vi "GIS Error Monitor Process.vi"(8 "error in":errorcluster, 9 "notifierSync":refnum<notifier>, 10 "TopLevel":refnum<class "TopLevel.lvclass">, 11 "GIS Printer in":refnum<class "GIS Printer.lvclass">) -> (3 "GIS Printer out":refnum<class "GIS Printer.lvclass">)   [LabVIEW 2022 SP3, in "GIS Printer.lvclass"]
uses:
  GIS Printer.lvclass
  TopLevel/TopLevel.lvclass
panel:
  out "error out":errorcluster
  in  "OK":bool
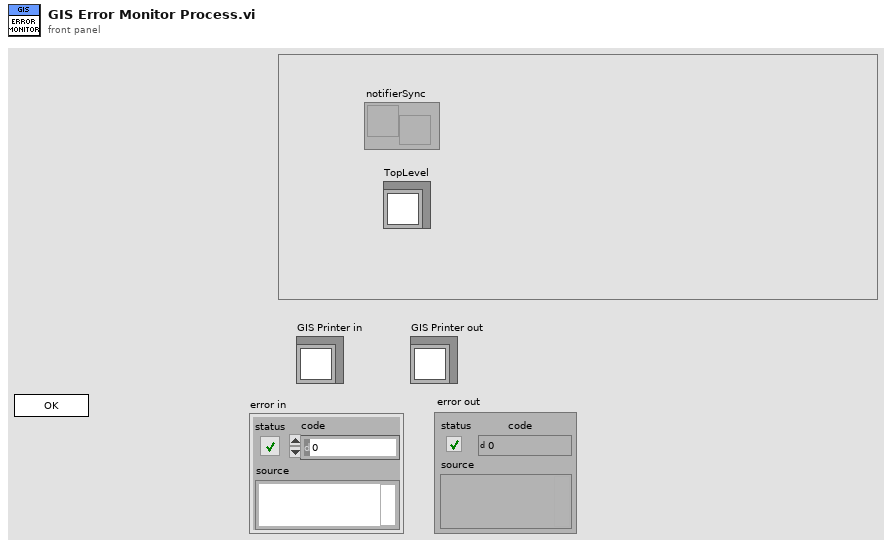
[diagram p1: front panel]
types:
  T1 = enum32{"invalid app kind", "Development System", "Run Time System", "Student Edition", "Embedded LabVIEW", "Evaluation", "Custom"}
  T2 = enum32{"Invalid", "Standard", "Closed", "Hidden", "Minimized", "Maximized"}
  T3 = cluster{"TimeStamp":timestamp, "Error":errorcluster}
  T4 = cluster{"Core":cluster{"Current VI Reference":refnum<vi>, "Close Panel on Exit?":bool}, "GIS Printer in":refnum<class "GIS Printer.lvclass">, "TO":i32, "notifierSync":refnum<notifier>}
  T5 = cluster{"Current VI Reference":refnum<vi>, "Close Panel on Exit?":bool}
  T6 = typedef "TopLevel.lvclass/UserEvents.ctl" = cluster{"API Incoming Event":refnum<user-event>, "API Executed Event":refnum<user-event>, "API Return Event":refnum<user-event>, "Exit Event":refnum<user-event>, "StatusChanged":refnum<user-event>, "DLP GUI Config Changed":refnum<user-event>, "AppEvent":refnum<user-event>, "Login Event":refnum<user-event>}
  T7 = typedef "GIS Printer.lvclass/UserEvents.ctl" = cluster{"API Incoming Event":refnum<user-event>, "API Executed Event":refnum<user-event>, "API Return Event":refnum<user-event>, "Status Changed Event":refnum<user-event>, "Abort":refnum<user-event>, "stop process":refnum<user-event>, "GISPollStatus":refnum<user-event>, "GISHeadStatus":refnum<user-event>, "Error Event":refnum<user-event>}
  T8 = enum16{"open", "replace", "create", "open or create", "replace or create", "replace or create with confirmation"}
  T9 = typedef "TD Pathnames--cluster.ctl" = cluster{"RunTimeSys?":bool, "AppFolder":path, "ExecutablePath":path, "ConfigFolder":path, "DataLogFolder":path, "SystemLogFolder":path, "SeqFolder":path, "MainStartupPathname":path, "MainUIPathname":path, "SystemEventsFile":path, "SeqEventsFile":path, "Config SettingsFile":path, "DAQ IOConfigFile":path, "SystemSimulation":bool, "DLPUIConfigFile":path, "PrinterInitXMLFile":path, "PersistentXMLFile":path, "Error Log Folder":path, "RecipeXMLFolder":path}
  T10 = cluster{"Log Data":string, "Current LogFile Name":string, "File Refnum":refnum<file>, "dup Directory Path":path}
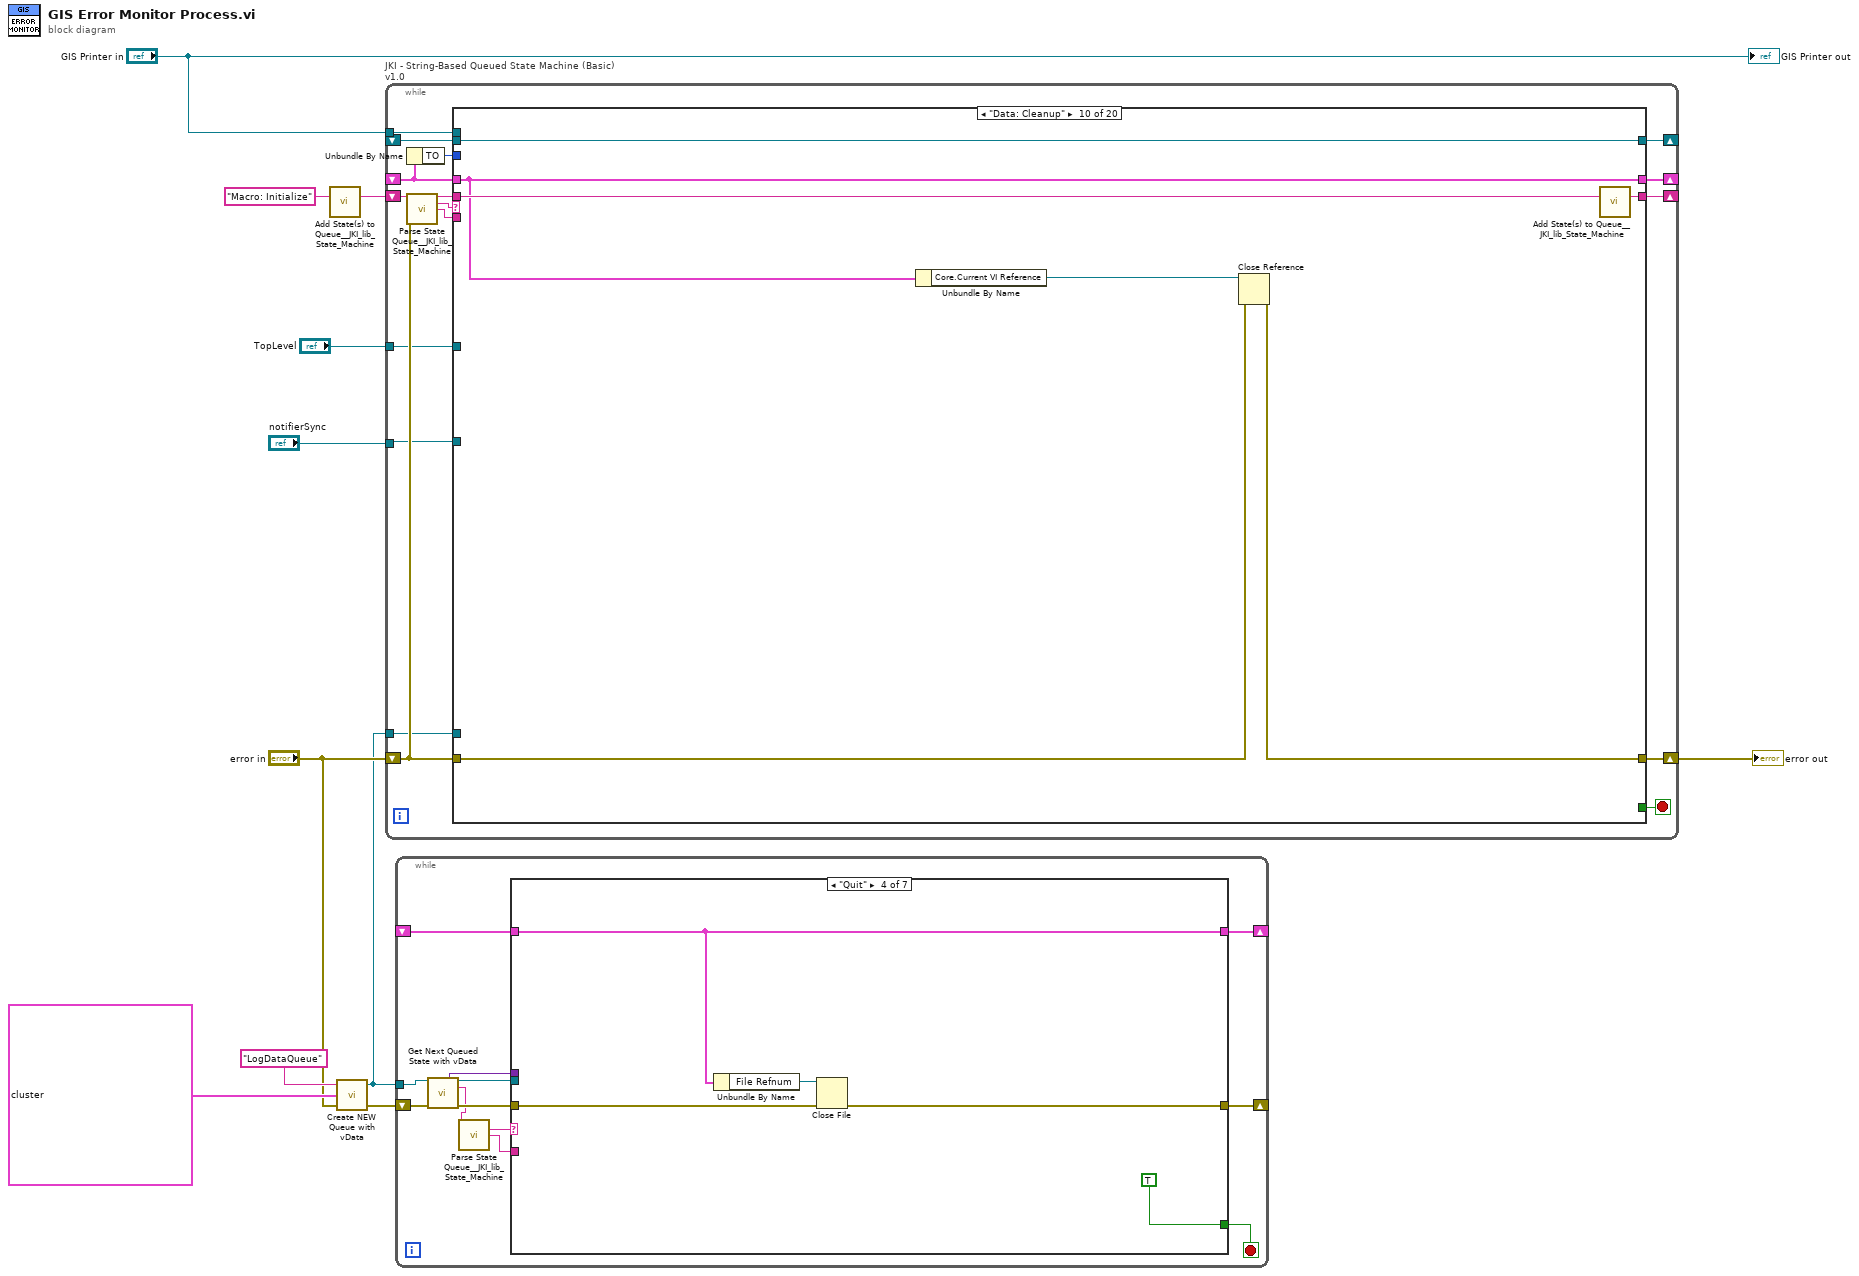
[diagram p0: block diagram]
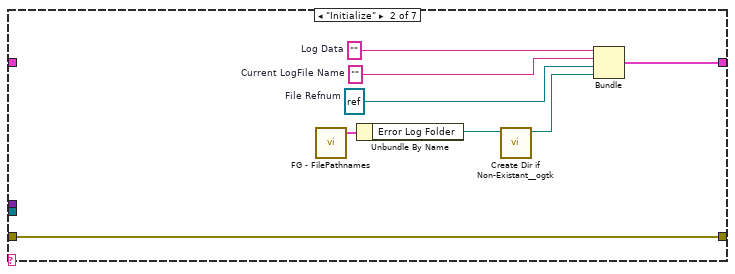
[diagram p3: hidden frame]
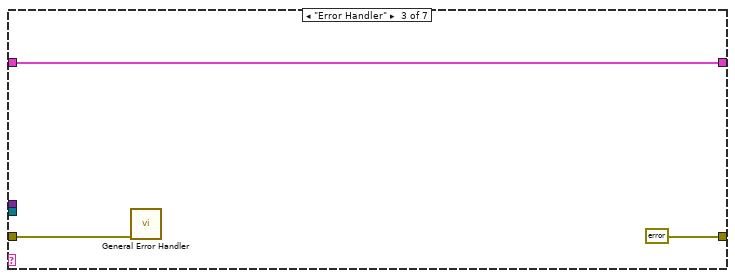
[diagram p4: hidden frame]
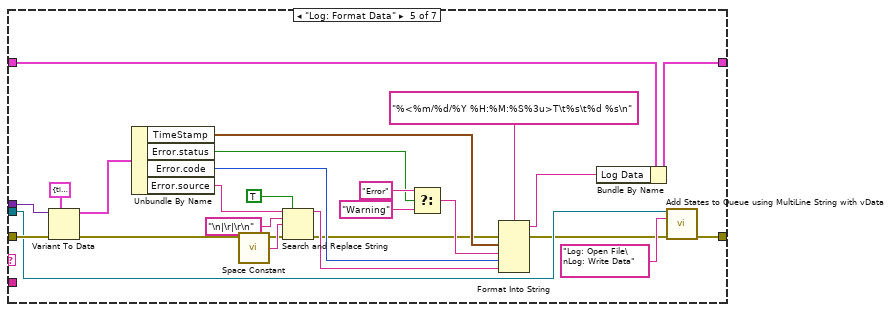
[diagram p5: hidden frame]
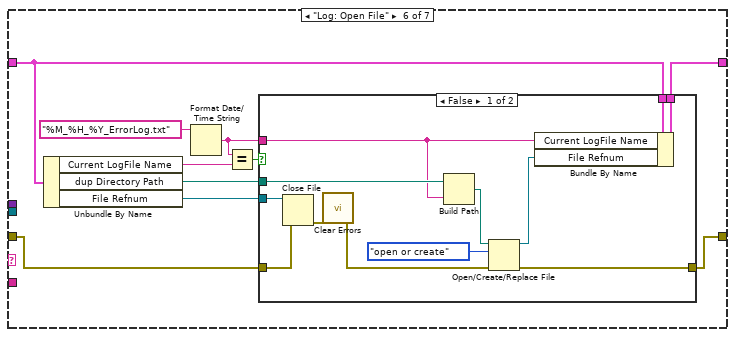
[diagram p6: hidden frame]
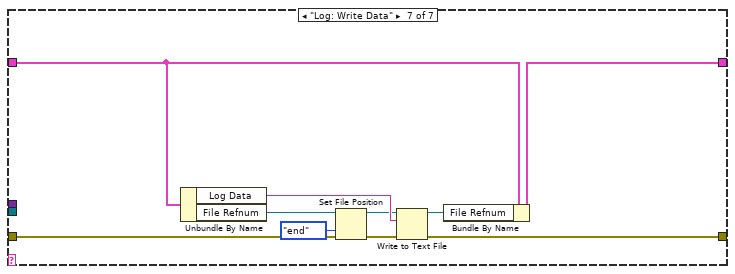
[diagram p8: hidden frame]
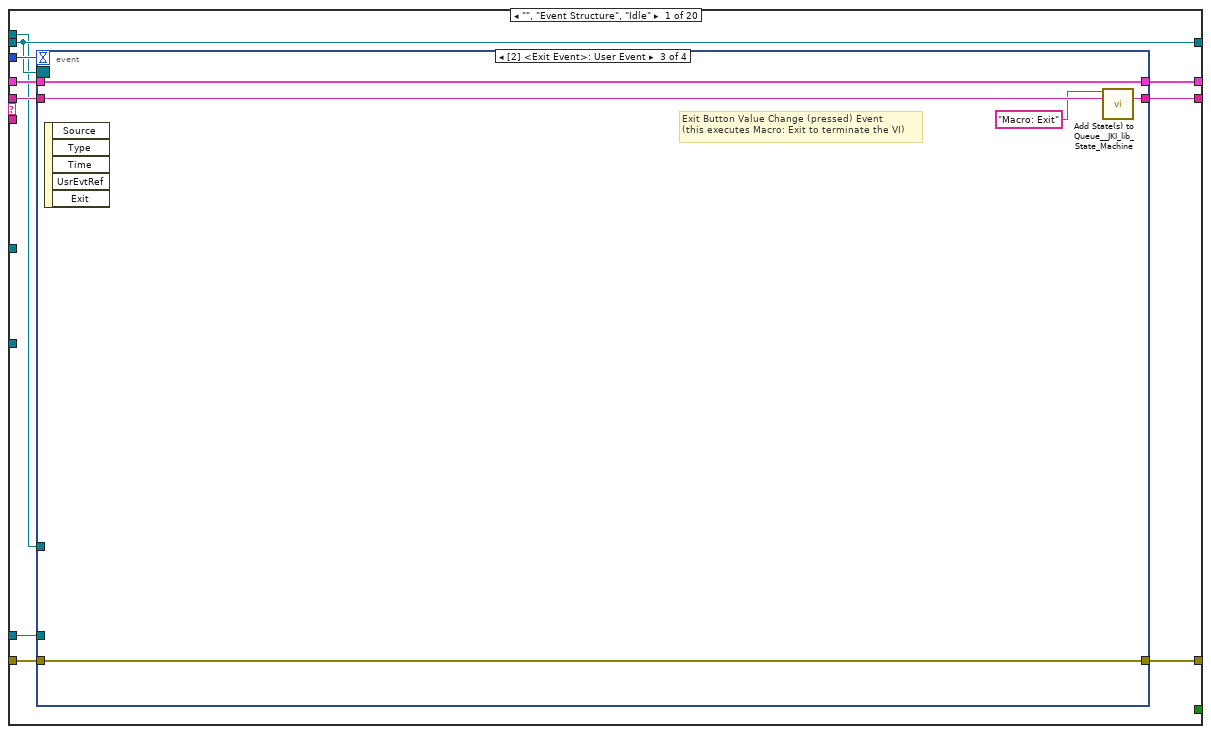
[diagram p9: hidden frame]
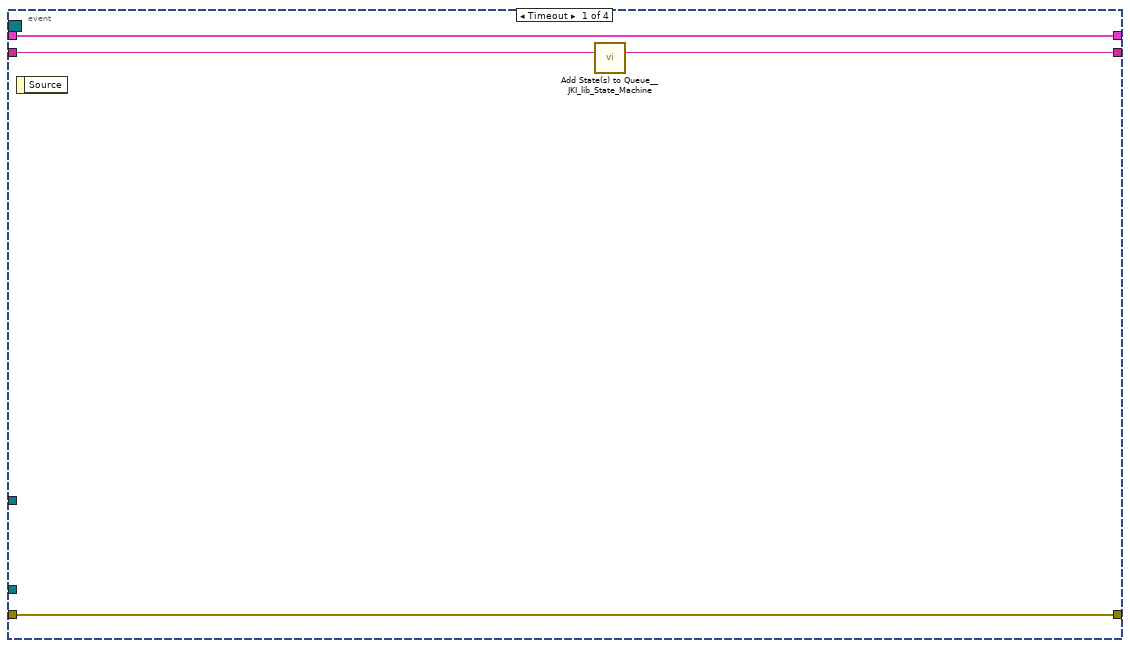
[diagram p10: hidden frame]
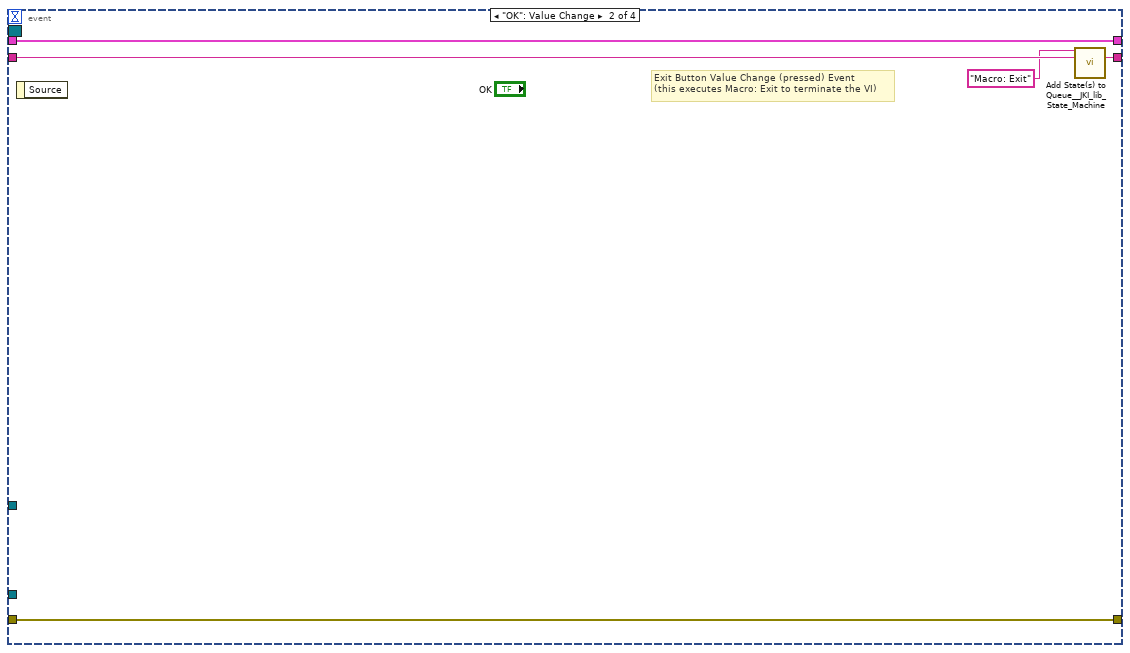
[diagram p11: hidden frame]
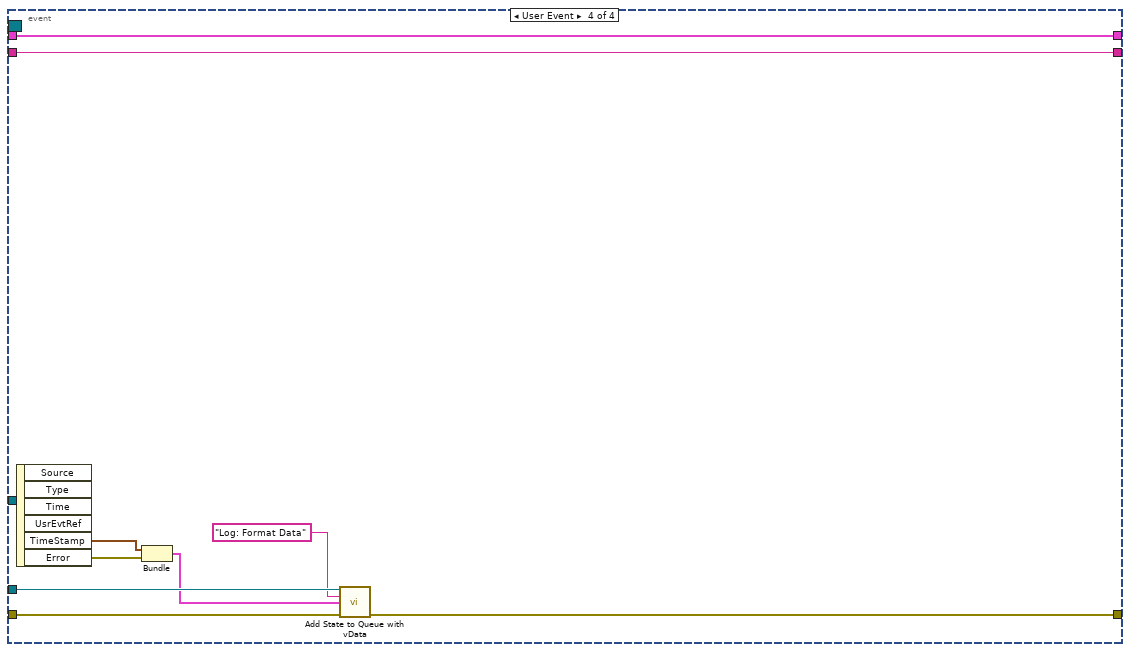
[diagram p12: hidden frame]
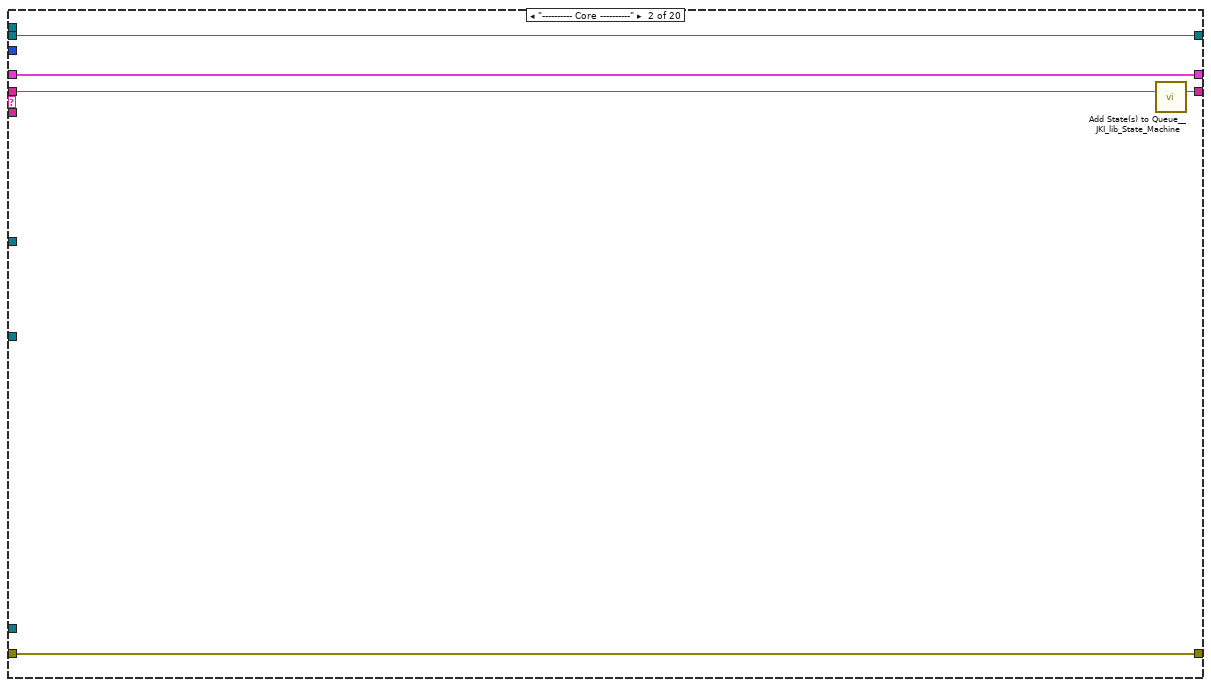
[diagram p13: hidden frame]
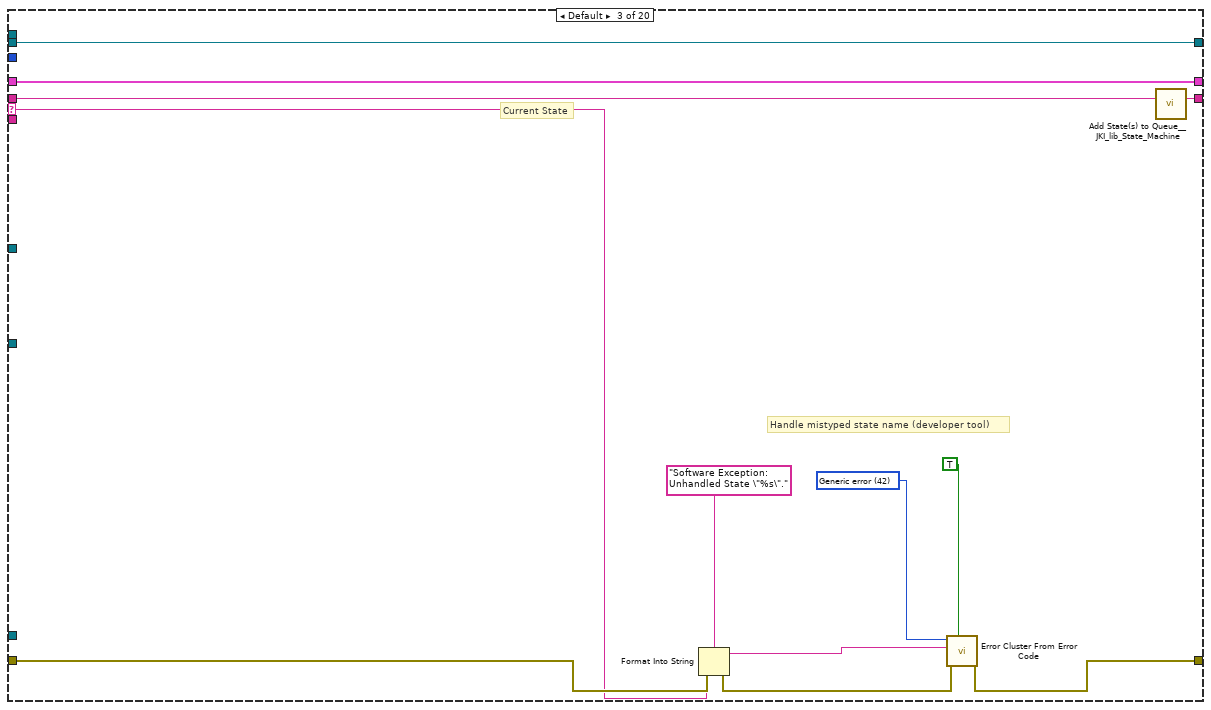
[diagram p14: hidden frame]
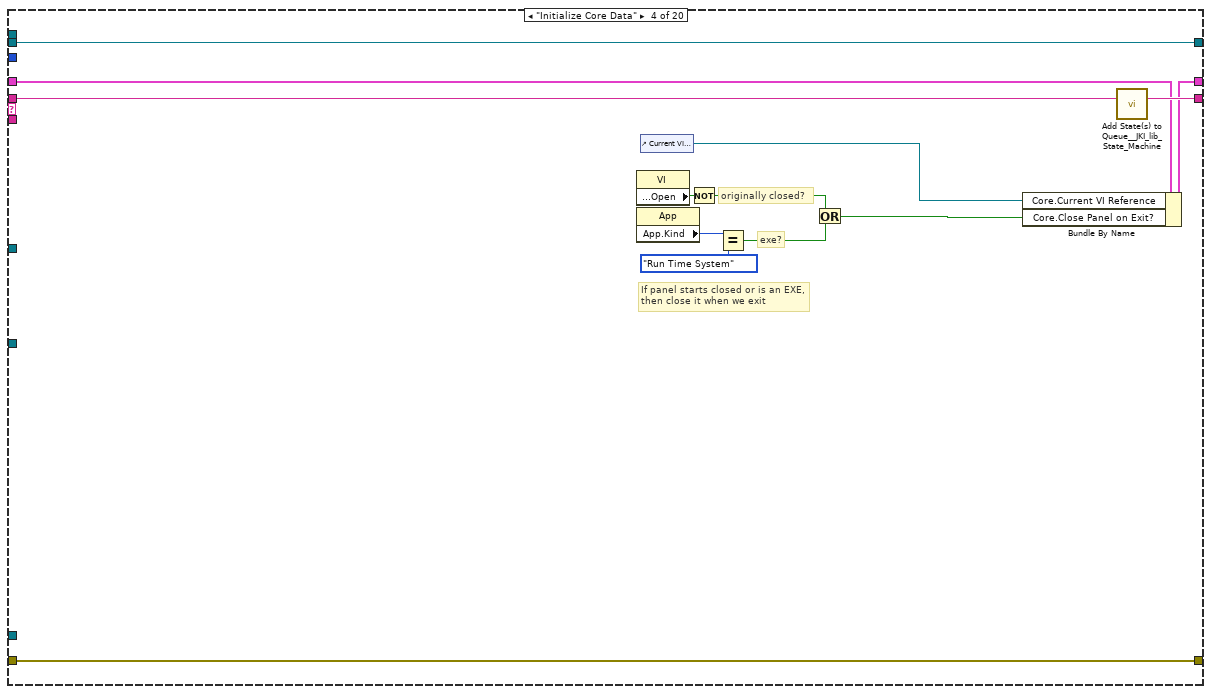
[diagram p15: hidden frame]
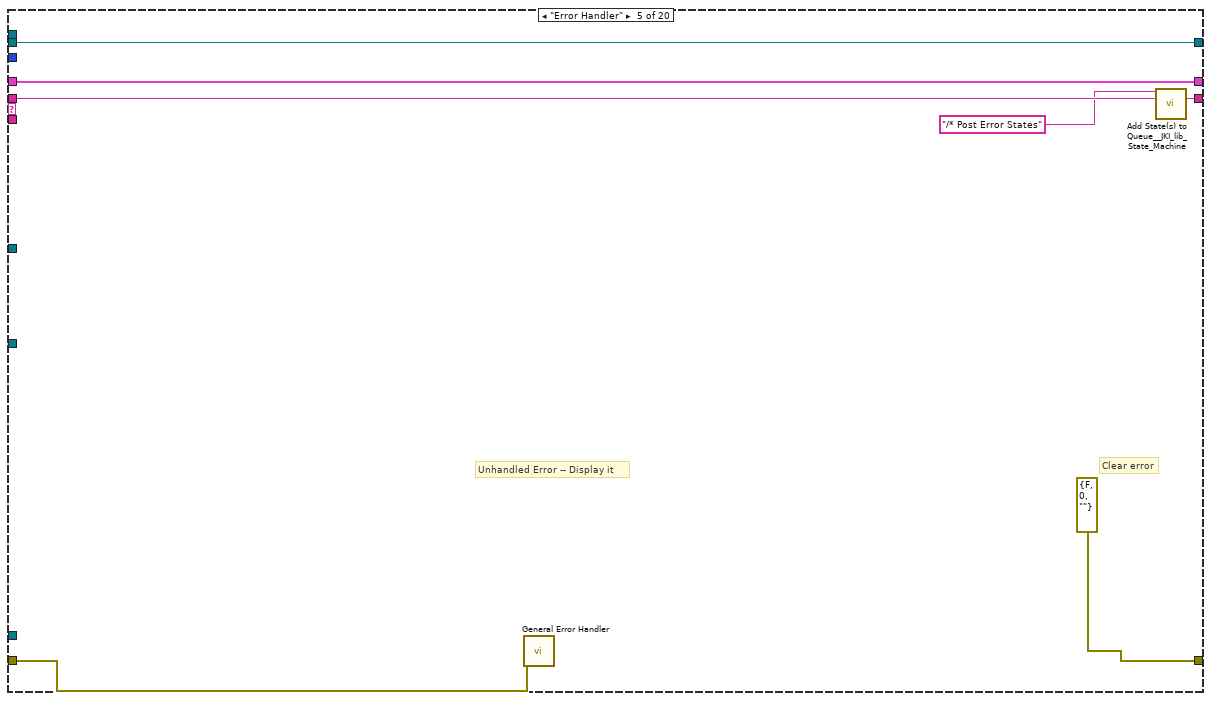
[diagram p16: hidden frame]
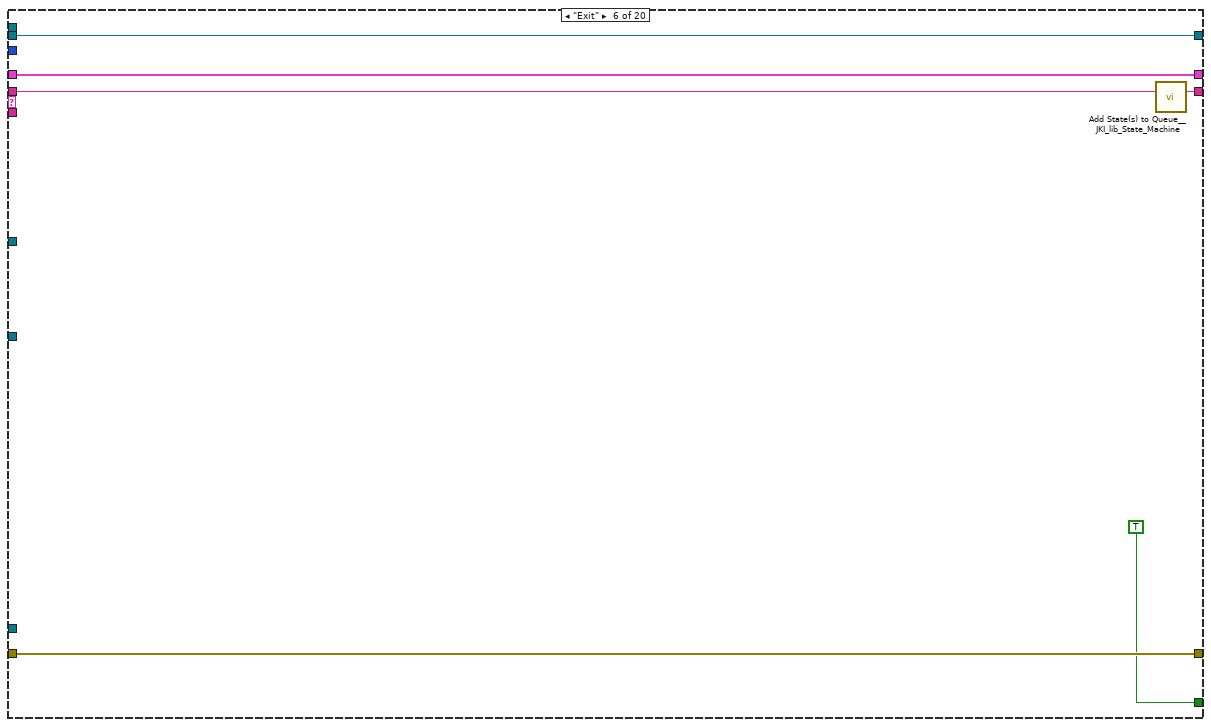
[diagram p17: hidden frame]
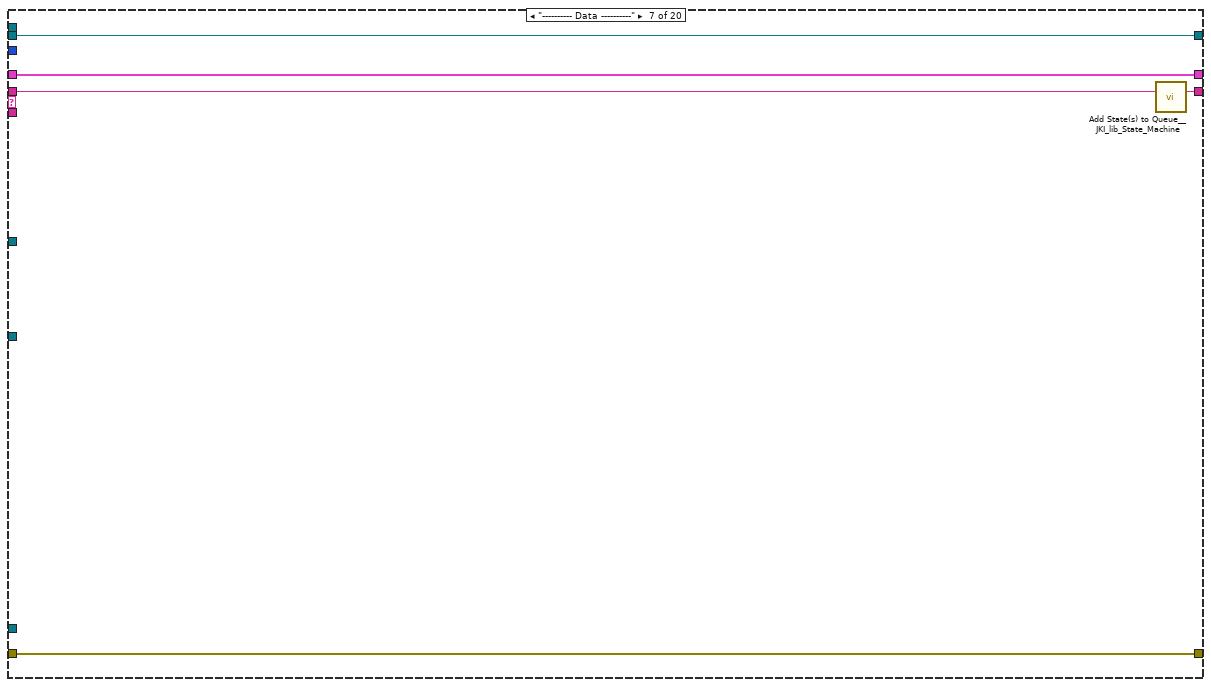
[diagram p18: hidden frame]
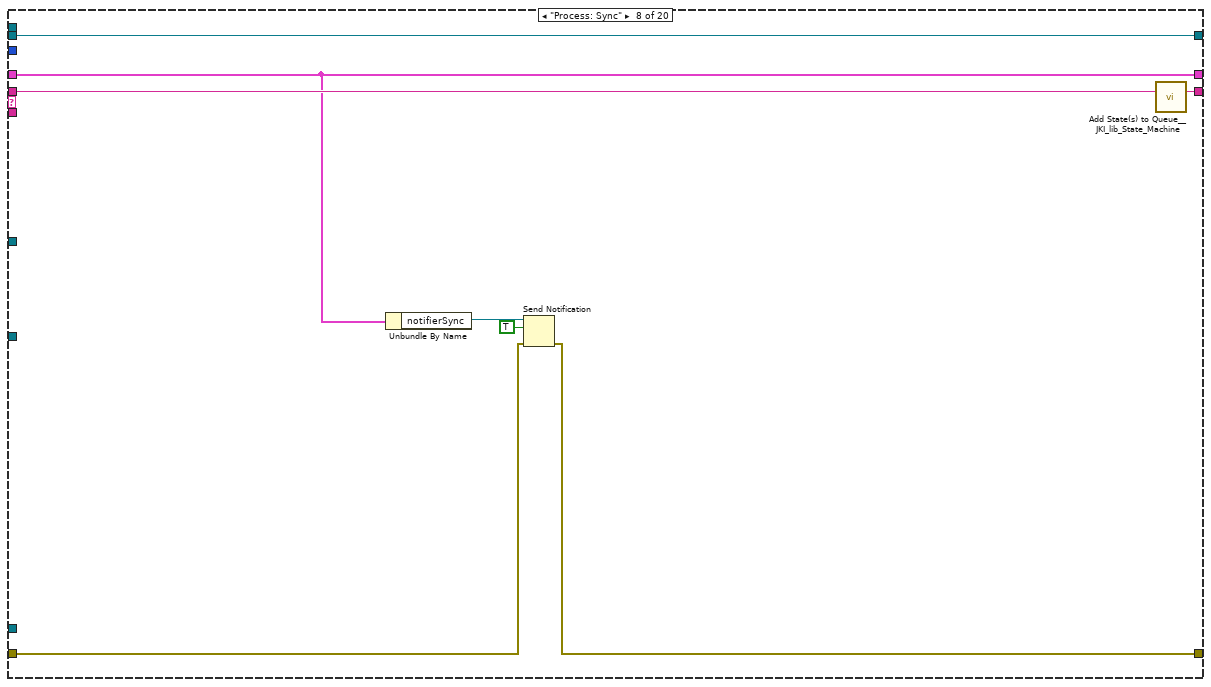
[diagram p19: hidden frame]
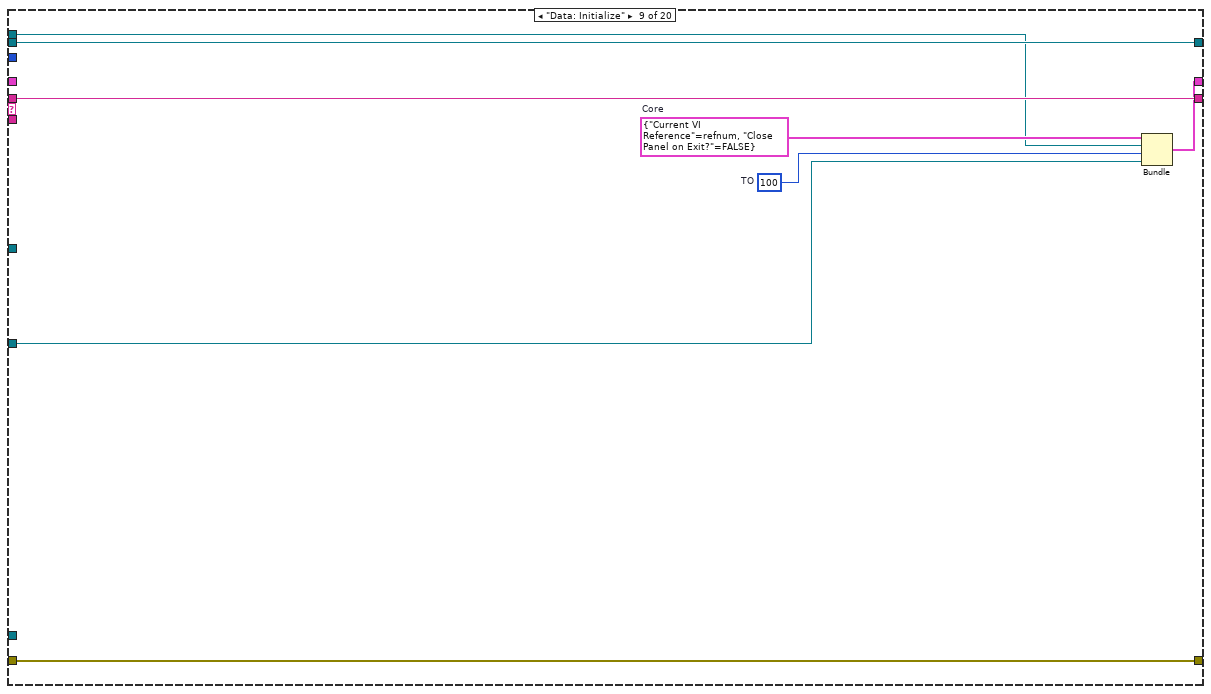
[diagram p20: hidden frame]
diagram:
  n1 = call <vilib>:"Add State(s) to Queue__JKI_lib_State_Machine.vi"("State(s) in (\"\")"="Macro: Initialize") -> ("States Out"=w11:string)  [unwired: 14 in]
  n2 = call <vilib>:"Create NEW Queue with vData.vi"("error in (no error)"="error in", "Initial States"=cluster{"state":string, "vData":variant}[] [{"state"="Initialize", "vData"=variant}, {"state"="Log: Open File", "vData"=variant}], "Name (SMQ)"="LogDataQueue") -> ("error out"=w4:errorcluster, "queue out"=w1:refnum<queue>)  [unwired: 1 in]
  n3 = while "JKI - String-Based Queued State Machine (Basic) v1.0" {
    shift-right: [w21] -> _
    shift-left: _ -> [w15]
    shift-right: [w24] -> w8
    shift-left: "error in" -> [w20]
    shift-right: [w23] -> _
    shift-left: w11 -> [w25]
    tunnel: "GIS Printer in" -> [w19]
    shift-right: [w18] -> _
    shift-left: _ -> [w17]
    tunnel: "TopLevel" -> [w14]
    tunnel: "notifierSync" -> [w13]
    tunnel: w1 -> [w12]
    stop <- w22 stop-if-true
    n4 = Unbundle By Name(w15) -> ("TO"=w16:i32)
    n5 = call <vilib>:"Parse State Queue__JKI_lib_State_Machine.vi"("State Queue"=w25, "Error In (no error)"=w20) -> ("Remaining States"=w27:string, "Current State"=w28:string, "Arguments"=w26:string)  [unwired: 11 in]
    n6 = case shown="\"Data: Cleanup\"" w28 {
      selector: w28 -> [_ _ w68 _ _ _ _ _ _ _ _ _ _ _ _ _ _ _ _ _]
      tunnel: w27 -> [w38 w66 w72 w91 w98 w104 w109 w117 w125 w132 w137 w143 w150 w162 w189 _ w207 w211 w224 w229]
      tunnel: w26 -> [_ _ _ _ _ _ _ _ _ _ _ _ w145 w156 _ _ _ _ _ _]
      tunnel: w15 -> [w36 w63 w70 w82 w95 w102 w106 w112 _ w128 w134 w141 w148 w158 w186 w191 w205 w209 w221 w228]
      tunnel: [w35 w64 w74 w88 errorcluster {"status"=FALSE, "code"=0, "source"=""} ("error out") w101 w107 w111 w118 w129 w135 w138 w146 w159 w187 w194 w195 w210 w219 w227] -> w24
      tunnel: w20 -> [w34 w64 w73 w88 w94 w101 w107 w110 w118 w126 w135 w139 w147 w160 w187 w194 _ w210 w212 w226]
      tunnel: [w37 w65 w71 w90 w97 w103 w108 w116 w125 w131 w136 w142 w149 w161 w188 w193 w206 w211 w223 w229] -> w23
      tunnel: [_ _ _ _ _ TRUE _ _ _ _ _ _ _ _ _ _ _ _ _ _] -> w22
      tunnel: [w33 w63 w70 w89 w95 w102 w106 w112 w124 w128 w134 w141 w148 w158 w186 w191 w205 w209 w221 w228] -> w21
      tunnel: w16 -> [w32 _ _ _ _ _ _ _ _ _ _ _ _ _ _ _ _ _ _ _]
      tunnel: w19 -> [w30 _ _ _ _ _ _ _ w120 _ _ _ _ _ _ _ _ _ _ _]
      tunnel: [w31 w62 w67 w79 w92 w99 w105 w115 w122 w127 w133 w140 w144 w155 w185 w190 w198 w208 w222 w225] -> w18
      tunnel: w17 -> [w31 w62 w67 w79 w92 w99 w105 w115 w122 w127 w133 w140 w144 w155 w185 w190 w198 w208 _ w225]
      tunnel: w14 -> [_ _ _ _ _ _ _ _ _ _ _ _ _ _ _ _ _ _ w215 _]
      tunnel: w13 -> [_ _ _ _ _ _ _ _ w119 _ _ _ _ _ _ _ _ _ _ _]
      tunnel: w12 -> [w29 _ _ _ _ _ _ _ _ _ _ _ _ _ _ _ w196 _ _ _]
      frame "", "Event Structure", "Idle" {
        n7 = event shown="[2] <Exit Event>: User Event" {
          selector: w31 -> [_ _ _ _]
          dyn-events: _ -> [_ _ _ _]
          timeout: w32 -> [_ _ _ _]
          tunnel: w38 -> [w42 w47 w52 w61]
          tunnel: [w41 w46 w51 w61] -> w37
          tunnel: w36 -> [w39 w44 w49 w60]
          tunnel: [w40 w45 w50 w53] -> w35
          tunnel: w34 -> [w40 w45 w50 w54]
          tunnel: [w39 w44 w49 w60] -> w33
          tunnel: w30 -> [_ _ _ _]
          tunnel: w29 -> [_ _ _ w59]
          event Timeout {
            n8 = event-data() -> ()  [unwired: 1 in, 1 out]
            n9 = call <vilib>:"Add State(s) to Queue__JKI_lib_State_Machine.vi"("State(s) in (\"\")"=w42) -> ("States Out"=w41:string)  [unwired: 14 in]
          }
          event "OK": Value Change {
            # "Exit Button Value Change (pressed) Event\n(this executes Macro: Exit to terminate the VI)"
            n10 = event-data() -> ()  [unwired: 1 in, 1 out]
            n11 = call <vilib>:"Add State(s) to Queue__JKI_lib_State_Machine.vi"("State(s) in Front (\"\")"="Macro: Exit", "State(s) in (\"\")"=w47) -> ("States Out"=w46:string)  [unwired: 13 in]
          }
          event User Event {
            # "Exit Button Value Change (pressed) Event\n(this executes Macro: Exit to terminate the VI)"
            n12 = event-data() -> ()  [unwired: 1 in, 5 out]
            n13 = call <vilib>:"Add State(s) to Queue__JKI_lib_State_Machine.vi"("State(s) in Front (\"\")"="Macro: Exit", "State(s) in (\"\")"=w52) -> ("States Out"=w51:string)  [unwired: 13 in]
          }
          event User Event {
            n14 = event-data() -> ("TimeStamp"=w57:timestamp, "Error"=w56:errorcluster)  [unwired: 1 in, 4 out]
            n15 = Bundle("TimeStamp"=w57, "Error"=w56) -> (w55:T3)  [unwired: 1 in]
            n16 = call <vilib>:"Add State to Queue with vData.vi"("queue in"=w59, "state in"="Log: Format Data" ("states in"), "vData (\"\")"=w55, "error in"=w54) -> ("error out"=w53:errorcluster)  [unwired: 8 in, 3 out]
          }
        }
      }
      frame "---------- Core ----------" {
        n17 = call <vilib>:"Add State(s) to Queue__JKI_lib_State_Machine.vi"("State(s) in (\"\")"=w66) -> ("States Out"=w65:string)  [unwired: 14 in]
      }
      frame Default {
        w77 = 42 items=["No error", "Argument error", "Memory is full", "Out of zone", "End of file", "File already open", "Generic file I/O error", "File not found", "File permission error", "Disk is full", "Duplicate path", "Too many files open", "System feature not enabled", "Resource file not found", "Cannot add resource", "Resource not found", "Image not found", "Image memory error", "Pen does not exist", "Config type invalid", "Config token not found", "Config parse error", "Config memory error", "Bad external code format", "Bad external code offset", "External code not present", "Null window", "Destroy window error", "Null menu", "Print aborted", "Bad print record", "Print driver error", "Windows error during printing", "Memory error during printing", "Print dialog error", "Generic print error", "Invalid device refnum", "Device not found", "Device parameter error", "Device unit error", "Cannot open device", "Device call aborted", "Generic error", "Cancelled by user", "Object ID too low", "Object ID too high", "Object not in heap", "Unknown heap", "Unknown object (invalid DefProc)", "Unknown object (DefProc not in table)", "Message out of range", "Invalid (null) method", "Unknown message", "Manager call not supported", "Bad address", "Network operation in progress", "Network operation timed out", "Connection is busy", "Network attribute not supported", "Network error", "Address in use", "System out of memory", "Connection aborted", "Connection refused", "Not connected", "Already connected", "Connection closed", "Initialization error (interapplication manager)", "Bad occurrence", "Wait on unbound occurrence handler", "Occurrence queue overflow", "Datalog type conflict", "Unused", "Unrecognized type (interapplication manager)", "Memory corrupt", "Failed to make temporary DLL", "Old CIN version", "Drag socket not found", "Failed to load drop-object", "Failed to register OLE object", "Failed to release OLE object", "Format specifier type mismatch", "Unknown format specifier", "Too few format specifiers", "Too many format specifiers", "Scan failed", "Newer CIN version", "Error converting to variant", "Runtime menu error", "Password tampered", "Variant attribute not found", "Incompatible variant data type", "Event data is not available", "Event Store is not present", "Occurrence is not found", "Event Queue is not created", "Event info is not available", "Refnum passed is NULL", "Error retrieving Class GUID", "Error retrieving CoClass GUID", "Error retrieving TypeLib GUID.", "Bad built application magic bytes.", "Specific driver is different from the specific driver associated with the Logical Name.", "There is no session opened to the class driver.", "Max Error", "MAX - Error with config objects", "MAX - Error loading configuration", "MAX - Group not supported"]
        # "Current State"
        # "Handle mistyped state name (developer tool)"
        n18 = Format Into String(format string="Software Exception: Unhandled State \"%s\"." ("message"), error in=w73, w68) -> (resulting string=w76:string, error out=w75:errorcluster)  [unwired: 1 in]
        n19 = call <vilib>:"Error Cluster From Error Code.vi"("show call chain? (False)"=TRUE, "error in (no error)"=w75, "error message (\"\")"=w76, "error code (0)"=w77) -> ("error out"=w74:errorcluster)  [unwired: 5 in]
        n20 = call <vilib>:"Add State(s) to Queue__JKI_lib_State_Machine.vi"("State(s) in (\"\")"=w72) -> ("States Out"=w71:string)  [unwired: 14 in]
      }
      frame "Initialize Core Data" {
        # "originally closed?"
        # "exe?"
        # "If panel starts closed or is an EXE, then close it when we exit"
        n21 = property class="VI"() -> ("Front Panel.Open"=w87:bool)  [unwired: 2 in, 2 out]
        n22 = property class="App"() -> ("App.Kind"=w86:T1)  [unwired: 2 in, 2 out]
        n23 = control-ref of="Current VI Reference"() -> (w80:refnum<vi>)
        n24 = Not(x=w87) -> (.not. x?=w84:bool)
        n25 = Equal?(x=w86, y=T1."Run Time System" ("Application:Kind")) -> (x = y?=w83:bool)
        n26 = Or(x=w84, y=w83) -> (x .or. y?=w81:bool)
        n27 = Bundle By Name(cluster=w82, "Core.Current VI Reference"=w80, "Core.Close Panel on Exit?"=w81) -> (w89:T4)
        n28 = call <vilib>:"Add State(s) to Queue__JKI_lib_State_Machine.vi"("State(s) in (\"\")"=w91) -> ("States Out"=w90:string)  [unwired: 14 in]
      }
      frame "Error Handler" {
        # "Unhandled Error -- Display it"
        # "Clear error"
        n29 = call <vilib>:"General Error Handler.vi"("error in (no error)"=w94) -> ()  [unwired: 10 in, 5 out]
        n30 = call <vilib>:"Add State(s) to Queue__JKI_lib_State_Machine.vi"("State(s) in Front (\"\")"="/* Post Error States", "State(s) in (\"\")"=w98) -> ("States Out"=w97:string)  [unwired: 13 in]
      }
      frame "Exit" {
        n31 = call <vilib>:"Add State(s) to Queue__JKI_lib_State_Machine.vi"("State(s) in (\"\")"=w104) -> ("States Out"=w103:string)  [unwired: 14 in]
      }
      frame "---------- Data ----------" {
        n32 = call <vilib>:"Add State(s) to Queue__JKI_lib_State_Machine.vi"("State(s) in (\"\")"=w109) -> ("States Out"=w108:string)  [unwired: 14 in]
      }
      frame "Process: Sync" {
        n33 = Unbundle By Name(w112) -> ("notifierSync"=w114:refnum<notifier>)
        n34 = Send Notification(notification=TRUE, notifier=w114, error in (no error)=w110) -> (error out=w111:errorcluster)  [unwired: 1 out]
        n35 = call <vilib>:"Add State(s) to Queue__JKI_lib_State_Machine.vi"("State(s) in (\"\")"=w117) -> ("States Out"=w116:string)  [unwired: 14 in]
      }
      frame "Data: Initialize" {
        w121 = 100  # TO
        w123 = T5 {"Current VI Reference"=refnum, "Close Panel on Exit?"=FALSE}  # Core
        n36 = Bundle("Core"=w123, "GIS Printer in"=w120, "TO"=w121, "notifierSync"=w119) -> (w124:T4)  [unwired: 1 in]
      }
      frame "Data: Cleanup" {
        n37 = Unbundle By Name(w128) -> ("Core.Current VI Reference"=w130:refnum<vi>)
        n38 = Close Reference(reference=w130, error in (no error)=w126) -> (error out=w129:errorcluster)
        n39 = call <vilib>:"Add State(s) to Queue__JKI_lib_State_Machine.vi"("State(s) in (\"\")"=w132) -> ("States Out"=w131:string)  [unwired: 14 in]
      }
      frame "---------- UI ----------" {
        n40 = call <vilib>:"Add State(s) to Queue__JKI_lib_State_Machine.vi"("State(s) in (\"\")"=w137) -> ("States Out"=w136:string)  [unwired: 14 in]
      }
      frame "UI: Initialize" {
        n41 = call <userlib>:"Fit VI window to Largest Dec__ogtk.vi"("error in (no error)"=w139) -> ("error out"=w138:errorcluster)  [unwired: 5 in, 1 out]
        n42 = call <vilib>:"Add State(s) to Queue__JKI_lib_State_Machine.vi"("State(s) in (\"\")"=w143) -> ("States Out"=w142:string)  [unwired: 14 in]
      }
      frame "UI: Cursor Set" {
        # "Argument"
        n43 = case shown="\"Idle\", Default" w145 {
          tunnel: w147 -> [w152 w154]
          tunnel: [w151 w153] -> w146
          frame "Idle", Default {
            n44 = call <vilib>:"Unset Busy.vi"("error in (no error)"=w152) -> ("error out"=w151:errorcluster)  [unwired: 10 in]
          }
          frame "Busy" {
            n45 = call <vilib>:"Set Busy.vi"("error in (no error)"=w154) -> ("error out"=w153:errorcluster)  [unwired: 9 in, 1 out]
          }
        }
        n46 = call <vilib>:"Add State(s) to Queue__JKI_lib_State_Machine.vi"("State(s) in (\"\")"=w150) -> ("States Out"=w149:string)  [unwired: 14 in]
      }
      frame "UI: Front Panel State" {
        # "Argument"
        n47 = Unbundle By Name(w158) -> ("Core.Current VI Reference"=w157:refnum<vi>)
        n48 = case shown="\"Open\", Default" w156 {
          tunnel: w160 -> [w166 w179]
          tunnel: [w168 w180] -> w159
          tunnel: w157 -> [w167 w177]
          frame "Open", Default {
            n49 = property class="VI"(reference=w167, error in=w166) -> (reference out=w164:refnum<vi>, error out=w165:errorcluster, "Front Panel.Open"=w163:bool)
            n50 = case shown="False" w163 {
              tunnel: [w171 w174] -> w168
              tunnel: w165 -> [w170 w174]
              tunnel: w164 -> [w169 _]
              frame False {
                n51 = invoke class="VI" method="FP.Open"(reference=w169, error in=w170, "Activate"=TRUE, "State"=T2."Standard") -> (error out=w171:errorcluster)  [unwired: 1 in, 4 out]
              }
              frame True {
              }
            }
          }
          frame "Close" {
            n52 = property class="VI"(reference=w177, error in=w179) -> (reference out=w176:refnum<vi>, error out=w178:errorcluster, "Front Panel.Open"=w175:bool)
            n53 = case shown="True" w175 {
              tunnel: [w181 w184] -> w180
              tunnel: w178 -> [w181 w183]
              tunnel: w176 -> [_ w182]
              frame False {
              }
              frame True {
                n54 = invoke class="VI" method="FP.Close"(reference=w182, error in=w183) -> (error out=w184:errorcluster)  [unwired: 1 in, 2 out]
              }
            }
          }
        }
        n55 = call <vilib>:"Add State(s) to Queue__JKI_lib_State_Machine.vi"("State(s) in (\"\")"=w162) -> ("States Out"=w161:string)  [unwired: 14 in]
      }
      frame "---------- Macro ----------" {
        n56 = call <vilib>:"Add State(s) to Queue__JKI_lib_State_Machine.vi"("State(s) in (\"\")"=w189) -> ("States Out"=w188:string)  [unwired: 14 in]
      }
      frame "Macro: Initialize" {
        w192 = "Data: Initialize\nInitialize Core Data\nUI: Initialize\nEvents: Register Events\nProcess: Sync\n/*UI: Front Panel State >> Open"  # Data: Initialize Initialize Core Data UI: Initialize Events: Register Events Process: Sync /*UI: Front Panel State >> Open
        n57 = call <vilib>:"Add State(s) to Queue__JKI_lib_State_Machine.vi"("State(s) in (\"\")"=w192) -> ("States Out"=w193:string)  [unwired: 14 in]
      }
      frame "Macro: Exit" {
        n58 = call <vilib>:"Add State to Queue with vData.vi"("queue in"=w196, "state in"="Quit" ("states in")) -> ("error out"=w195:errorcluster)  [unwired: 10 in, 3 out]
        n59 = Unbundle By Name(w205) -> ("Core.Close Panel on Exit?"=w204:bool)
        n60 = Select(t="UI: Front Panel State >> Close", s=w204, f="") -> (s? t:f=w201:string)
        n61 = call <vilib>:"Add State(s) to Queue__JKI_lib_State_Machine.vi"("State(s) in (\"\")"=w201, "State(s) at Back (\"\")"="Data: Cleanup\nEvents: Unregister Events\nExit") -> ("States Out"=w199:string)  [unwired: 13 in]
        n62 = call <vilib>:"Add State(s) to Queue__JKI_lib_State_Machine.vi"("State(s) in Front (\"\")"=w199, "State(s) in (\"\")"=w207) -> ("States Out"=w206:string)  [unwired: 13 in]
      }
      frame "---------- Events ----------" {
      }
      frame "Events: Register Events" {
        n63 = call-dynamic "GetEvents_TopLevel.vi"("error in (no error)"=w212, "TopLevel in"=w215) -> ("error out"=w213:errorcluster, "UserEvents"=w216:T6)  [unwired: 7 in, 1 out]
        n64 = Unbundle By Name(w216) -> ("Exit Event"=w214:refnum<user-event>)
        n65 = Unbundle By Name(w221) -> ("GIS Printer in"=w220:refnum<class "GIS Printer.lvclass">)
        n66 = call-dynamic "GetEvents_GIS Printer.vi"("error in (no error)"=w213, "TopLevel in"=w220) -> ("error out"=w219:errorcluster, "UserEvents"=w218:T7)  [unwired: 7 in, 1 out]
        n67 = Unbundle By Name(w218) -> ("Error Event"=w217:refnum<user-event>)
        n68 = register-events(w217, w214) -> (reference out=w222:refnum<event-registration>)  [unwired: 2 in, 1 out]
        n69 = call <vilib>:"Add State(s) to Queue__JKI_lib_State_Machine.vi"("State(s) in (\"\")"=w224) -> ("States Out"=w223:string)  [unwired: 14 in]
      }
      frame "Events: Unregister Events" {
        n70 = Unregister For Events(event registration refnum=w225, error in=w226) -> (error out=w227:errorcluster)
      }
    }
  }
  "error out" <- w8
  n71 = while {
    tunnel: w1 -> [w234]
    shift-right: [w238] -> _
    shift-left: w4 -> [w240]
    shift-right: [w235] -> _
    shift-left: _ -> [w236]
    stop <- w241 stop-if-true
    n72 = call <vilib>:"Get Next Queued State with vData.vi"("queue in"=w234, "error in (no error)"=w240) -> ("vData out"=w237:variant, "queue out"=w230:refnum<queue>, "Next State"=w233:string, "error out"=w239:errorcluster)  [unwired: 7 in, 3 out]
    n73 = call <vilib>:"Parse State Queue__JKI_lib_State_Machine.vi"("State Queue"=w233) -> ("Current State"=w232:string, "Arguments"=w231:string)  [unwired: 12 in, 1 out]
    n74 = case shown="\"Quit\"" w232 {
      tunnel: [_ _ _ TRUE _ _ _] -> w241
      tunnel: w239 -> [w243 w251 w253 w255 w275 w288 w310]
      tunnel: [w243 w251 errorcluster {"status"=FALSE, "code"=0, "source"=""} ("error out") w256 w260 w287 w309] -> w238
      tunnel: w237 -> [_ _ _ _ w273 _ _]
      tunnel: w236 -> [w242 _ w252 w258 w284 w285 w311]
      tunnel: [w242 w249 w252 w258 w265 w286 w312] -> w235
      tunnel: w231 -> [_ _ _ _ _ _ _]
      tunnel: w230 -> [_ _ _ _ w262 _ _]
      frame Default {
      }
      frame "Initialize" {
        w246 = refnum<file> refnum  # File Refnum
        w247 = ""  # Current LogFile Name
        w248 = ""  # Log Data
        n75 = call "FG - FilePathnames.vi"() -> ("FilePaths out"=w250:T9)  [unwired: 4 in, 1 out]
        n76 = Unbundle By Name(w250) -> ("Error Log Folder"=w245:path)
        n77 = call <userlib>:"Create Dir if Non-Existant__ogtk.vi"("Directory Path"=w245) -> ("dup Directory Path"=w244:path)  [unwired: 8 in, 2 out]
        n78 = Bundle("Log Data"=w248, "Current LogFile Name"=w247, "File Refnum"=w246, "dup Directory Path"=w244) -> (w249:T10)  [unwired: 1 in]
      }
      frame "Error Handler" {
        n79 = call <vilib>:"General Error Handler.vi"("error in (no error)"=w253) -> ()  [unwired: 10 in, 5 out]
      }
      frame "Quit" {
        n80 = Unbundle By Name(w258) -> ("File Refnum"=w257:refnum<file>)
        n81 = Close File(refnum=w257, error in=w255) -> (error out=w256:errorcluster)  [unwired: 1 out]
      }
      frame "Log: Format Data" {
        n82 = Variant To Data(error in=w275, type=T3 {"TimeStamp"=timestamp(0 s since 1904-01-01), "Error"={"status"=FALSE, "code"=0, "source"=""}} ("output cluster"), Variant=w273) -> (data=w272:T3, error out=w267:errorcluster)
        n83 = Unbundle By Name(w272) -> ("TimeStamp"=w271:timestamp, "Error.status"=w270:bool, "Error.code"=w269:i32, "Error.source"=w268:string)
        n84 = call <vilib>:"Space Constant.vi"() -> ("String"=w277:string)
        n85 = Search and Replace String(replace all?=TRUE ("replace all? (F)"), input string=w268, search string="\n|\r|\r\n", replace string=w277, error in=w267) -> (result string=w276:string, error out=w266:errorcluster)  [unwired: 3 in, 2 out]
        n86 = Select(t="Error", s=w270, f="Warning") -> (s? t:f=w280:string)
        n87 = Format Into String(format string="%<%m/%d/%Y %H:%M:%S%3u>T\t%s\t%d %s\n" ("time format string (%c)"), error in=w266, w271, w280, w269, w276) -> (resulting string=w264:string, error out=w261:errorcluster)  [unwired: 1 in]
        n88 = Bundle By Name(cluster=w284, "Log Data"=w264) -> (w265:T10)
        n89 = call <vilib>:"Add States to Queue using MultiLine String with vData.vi"("queue in"=w262, "states in"="Log: Open File\nLog: Write Data", "error in"=w261) -> ("error out"=w260:errorcluster)  [unwired: 10 in, 2 out]
      }
      frame "Log: Open File" {
        n90 = Unbundle By Name(w285) -> ("Current LogFile Name"=w292:string, "dup Directory Path"=w290:path, "File Refnum"=w291:refnum<file>)
        n91 = Format Date/Time String(time format string (%c)="%M_%H_%Y_ErrorLog.txt") -> (date/time string=w294:string)  [unwired: 2 in]
        n92 = Equal?(x=w294, y=w292) -> (x = y?=w293:bool)
        n93 = case shown="False" w293 {
          tunnel: [w305 w307] -> w287
          tunnel: w285 -> [w304 w308]
          tunnel: w290 -> [w303 _]
          tunnel: [w302 w308] -> w286
          tunnel: w291 -> [w300 _]
          tunnel: w288 -> [w295 w307]
          tunnel: w294 -> [w297 _]
          frame False {
            n94 = Close File(refnum=w300, error in=w295) -> (error out=w299:errorcluster)  [unwired: 1 out]
            n95 = call <vilib>:"Clear Errors.vi"("error in (no error)"=w299) -> ("error out"=w296:errorcluster)  [unwired: 5 in, 1 out]
            n96 = Build Path(base path=w303, name or relative path=w297) -> (appended path=w301:path)
            n97 = Open/Create/Replace File(file path (use dialog)=w301, error in=w296, operation (0:open)=T8."open or create") -> (refnum out=w298:refnum<file>, error out=w305:errorcluster)  [unwired: 3 in, 1 out]
            n98 = Bundle By Name(cluster=w304, "Current LogFile Name"=w297, "File Refnum"=w298) -> (w302:T10)
          }
          frame True {
          }
        }
      }
      frame "Log: Write Data" {
        n99 = Unbundle By Name(w311) -> ("Log Data"=w318:string, "File Refnum"=w316:refnum<file>)
        n100 = Set File Position(refnum=w316, from (0:start)=enum16{"start", "end", "current"}."end", error in=w310) -> (refnum out=w314:refnum<file>, error out=w315:errorcluster)  [unwired: 1 in]
        n101 = Write to Text File(file (use dialog)=w314, text=w318, error in=w315) -> (refnum out=w317:refnum<file>, error out=w309:errorcluster)  [unwired: 1 in, 1 out]
        n102 = Bundle By Name(cluster=w311, "File Refnum"=w317) -> (w312:T10)
      }
    }
  }
  "GIS Printer out" <- "GIS Printer in"
